vi "CTE_Analysis_Suite_UIUCv0.7.vi"() -> ()   [LabVIEW 2012]
uses:
  <vilib>/Utility/file.llb/Read From Spreadsheet File (string).vi
  <vilib>/Utility/file.llb/Write To Spreadsheet File (string).vi
panel:
  out "fpath1":string=" "
  out "deleted portion":string[][](array[string])=[["Filename", "TempC", "TempError"]]
  in  "Reset":bool
  in  "stop":bool
  in  "Tab Control":T1(tab)
  in  "iCTEAS":bool
  in  "Manual Temp Edit":bool
  in  "Remove File for Analysis":bool
  in  "Get RT Platinum Const.":bool
  out "Temperature Data from Platinum saved to:":path=path "C:/Users/jonesza/My Documents/My Dropbox/KrivenResearch/Ellipsoid/Data/testdata/CTEAS_Output/Data_Temperatures.lvm"
  in  "RT Platinum Lattice Constant":dbl=3.92296 format="%#.6g"
  in  "Load Files":bool
  in  "Input File Directory Path":path=path "C:/Users/jonesza/My Documents/My Dropbox/KrivenResearch/Ellipsoid/Data/testdata"
  out "Data Loaded":bool
  in  "Temperature Data":i32(listbox)
  in  "Input File Type":enum32{"CSV File", "JADE File"}(radio)=enum."JADE File"
  out "CTERun Path":string="C:\\Users\\jonesza\\Documents\\My Dropbox\\KrivenResearch\\Ellipsoid\\CTEAS\\data"
  in  "Crystal Symmetry":string(combo)="Monoclinic"
  in  "Phase to be Analyzed":string(combo)=" "
  in  "Polynomial Fit Order":sgl=2.0 format="%#_1g"
  out "Saved":bool
  out "File Saved to:":string="C:\\Users\\jonesza\\My Documents\\My Dropbox\\KrivenResearch\\Ellipsoid\\Data\\testdata\\CTEAS_Output\\LPTest1.csv"
  in  "Lattice Parameter Filename":string="LPTest1"
  in  "Save Lattice Parameters":bool
  in  "View Lattice Parameters":bool
  in  "gamma":bool
  in  "beta":bool
  in  "alpha":bool
  in  "c":bool
  in  "b":bool
  in  "a":bool
  out "Step 1 Data Loaded":bool
  in  "Run Analysis":bool
  in  "Symmetry\nOverride":bool
  in  "High Temperature (C)":dbl=1700.0
  in  "Temperature Step":dbl=25.0
  in  "Low Temperature (C)":dbl=25.0
  out "Results Ready":bool
  in  "HKL or UVW.":enum32{"Radio Selection 1", "Radio Selection 2"}(radio)
  in  "LW":dbl
  in  "KV":dbl=1.0
  in  "HU":dbl
  out "HU 2":string="H"
  out "KV 2":string="K"
  out "LW 2":string="L"
  in  "Make 2D Figure":bool
  in  "Make hkl (or uvw) Expansion Plot":bool
  in  "2D Figure CSV File Name":string="2Dtestfile"
  in  "Make 2D Figure CSV File":bool
  in  "Make hkl (or uvw) Expansion CSV File":bool
  in  "hkl (or uvw) Expansion CSV Filename":string="hkltestfile2"
  in  "HKL or UVW":enum32{"Radio Selection 1", "Radio Selection 2"}(radio)
  in  "hu":dbl
  out "hu":string="H"
  in  "lw":dbl=1.0
  out "lw 2":string="L"
  in  "kv":dbl
  out "kv 2":string="K"
  in  "Make CSV File":bool
  in  "CSV File Name":string="testfile"
  in  "Make Eigenvalue Plot":bool
  in  "Make 3D Figure":bool
  in  "Figure Temperature (C)":dbl=1000.0
  in  "Make Movie":bool
  in  "Movie File Name":string="testmovie"
  in  "Movie FPS":dbl=4.0
  in  "Y":dbl=768.0
  in  "X":dbl=1024.0
  out "Step 2 Analysis Run":bool
  out "BUSY":bool
  in  "Get Results":bool
  # "CTE Analysis Suite UIUC v0.61"
  # "Coefficient of Thermal Expansion Analysis Suite\nVersion: 0.6.1-Build 1\nDeveloped by: \n\n                          Zachary A. Jones\n                          Pankaj Sarin, Ph. D.\n                          Ryan P. Haggerty, Ph. D.\n\nContact Information:\n\n                          Waltraud M. Kriven, Ph. D.\n                          The University of Illinois at Urbana-Champaign\n                          Office 105 Materials Science and Engineering Building\n                          1304 W. Green St., Urbana, IL 61801\n                          Phone: (217)333-5258\n                          Fax:       (217)333-2736\n                          Email:   kriven@illinois.edu\n\n\nThis software is the intellectual property of the University of Illinois at Urbana-Champaign.  Funding for this project was provided by the Air Force Office of Scientific Research under the following grant:\n\nFA9550-06-1-0386\n\nPlease use this reference for publications including CTEAS analyses:\n\nJones, Z. 2012, \"CTEAS - A GUI based program to calculate coefficients of thermal expansion of crystalline materials from high temperature powder X-ray diffraction\", 36th International Conference & Exposition on Advanced Ceramics and Composites, Daytona Beach, FL, Hilton Daytona Beach Resort and Ocean Center, p. 41."
  # "Temperature Ranges"
  # "Lattice Parameter File Output"
  # "Lattice Parameter Selection"
  # "Select a phase first!"
  # "NOTE:\nReference angle for eigenvectors relative to hkl or uvw vector."
  # "Size of figures (in Pixels)"
  # "x"
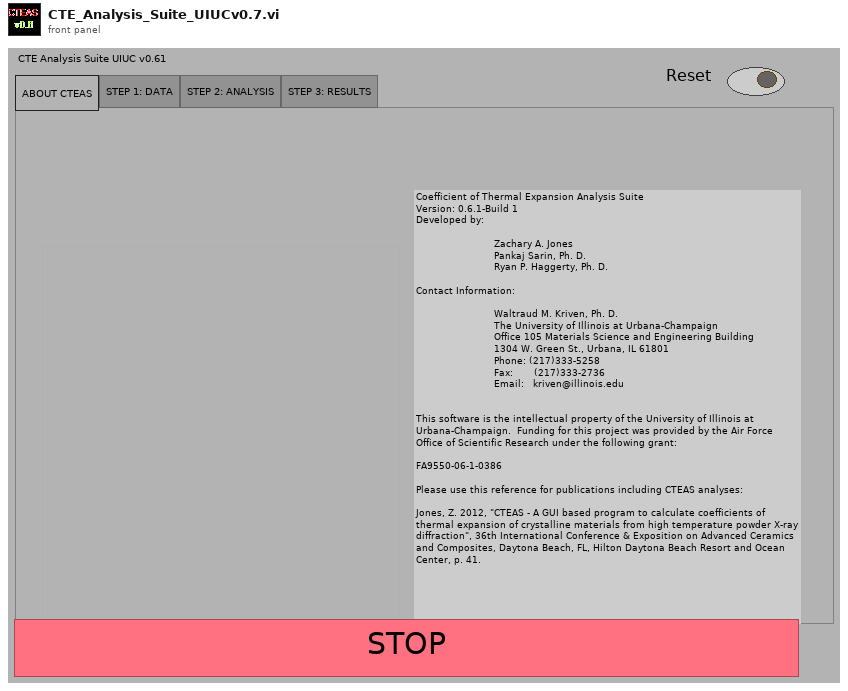
[diagram p1: front panel]
types:
  T1 = enum32{"ABOUT CTEAS", "STEP 1: DATA", "STEP 2: ANALYSIS", "STEP 3: RESULTS"}
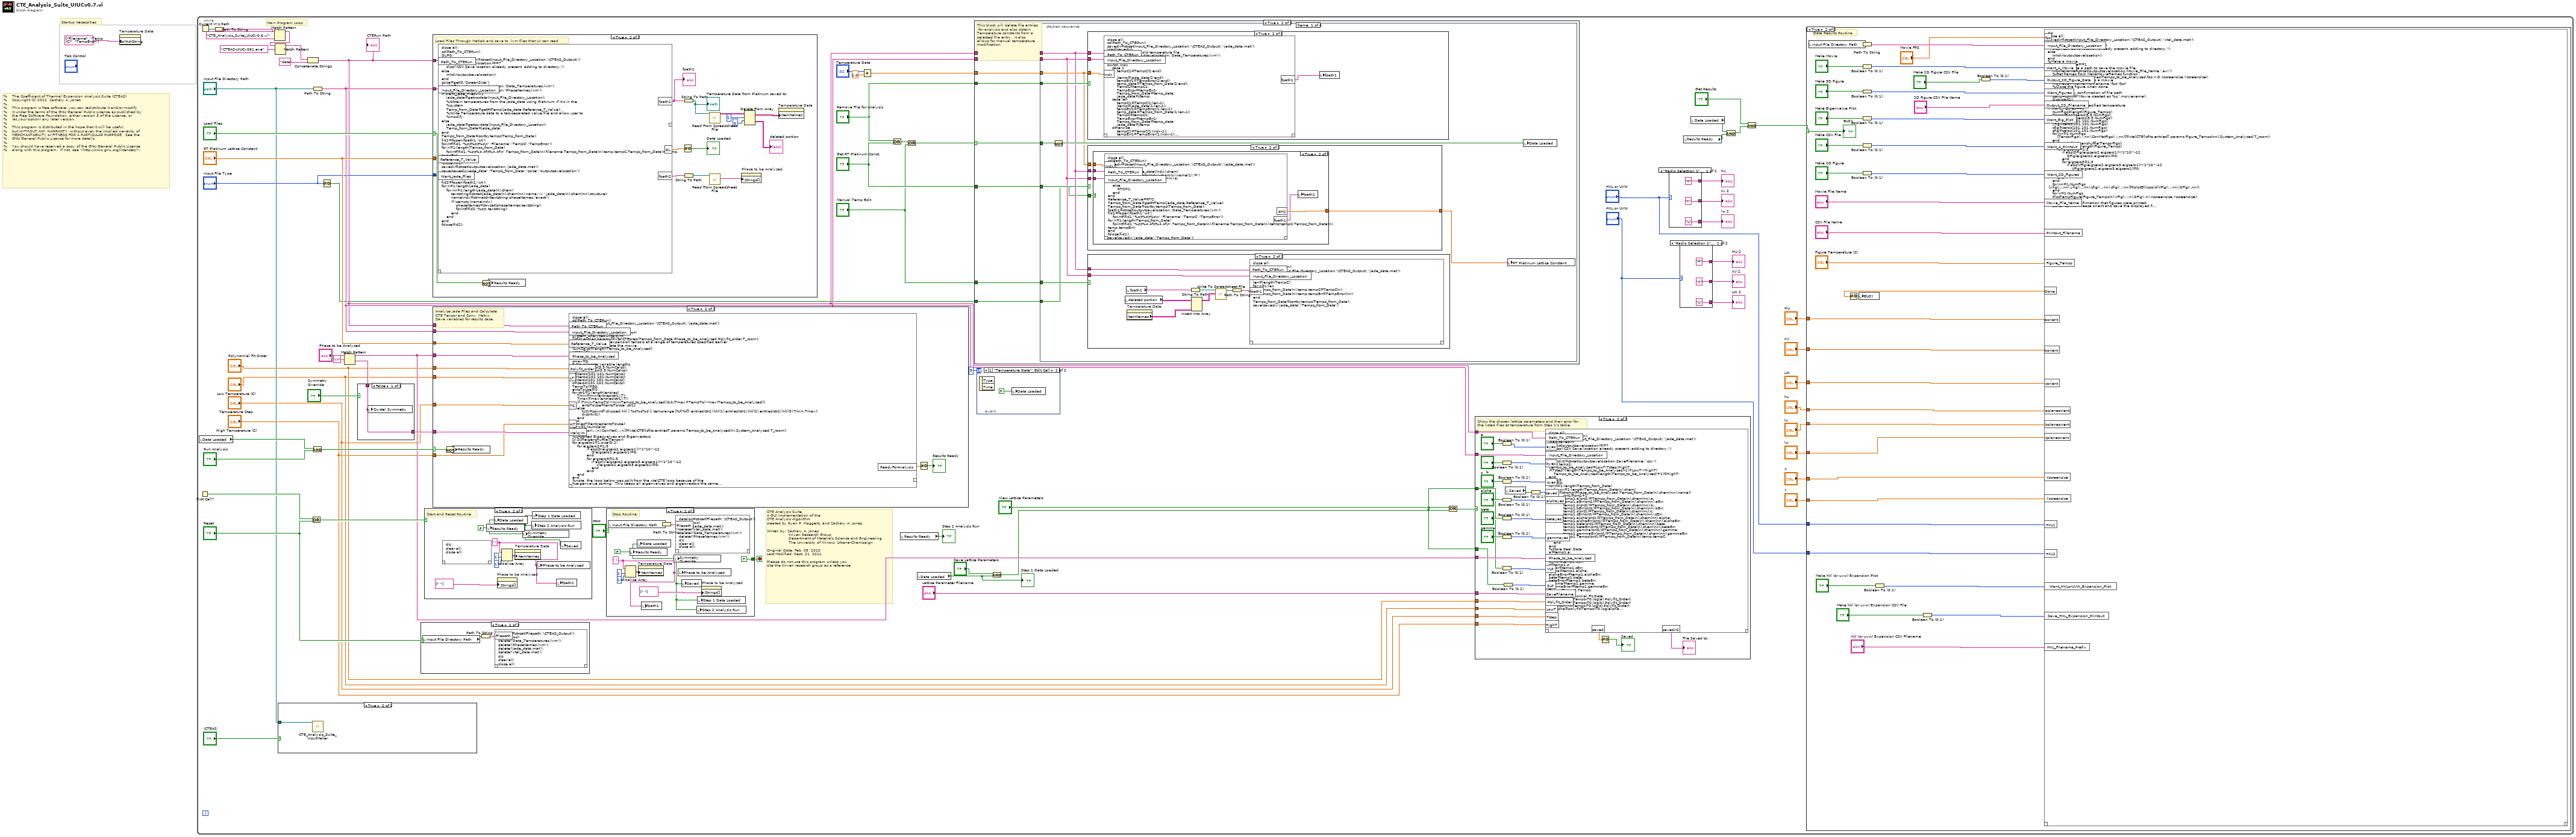
[diagram p0: block diagram]
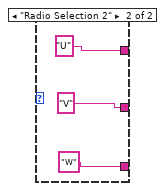
[diagram p3: hidden frame]
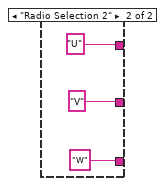
[diagram p4: hidden frame]
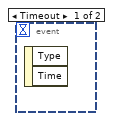
[diagram p7: hidden frame]
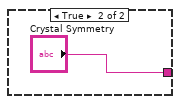
[diagram p8: hidden frame]
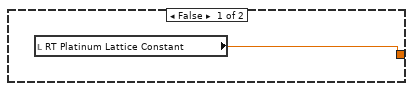
[diagram p11: hidden frame]
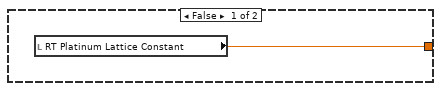
[diagram p12: hidden frame]
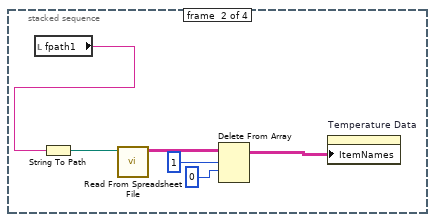
[diagram p14: hidden frame]
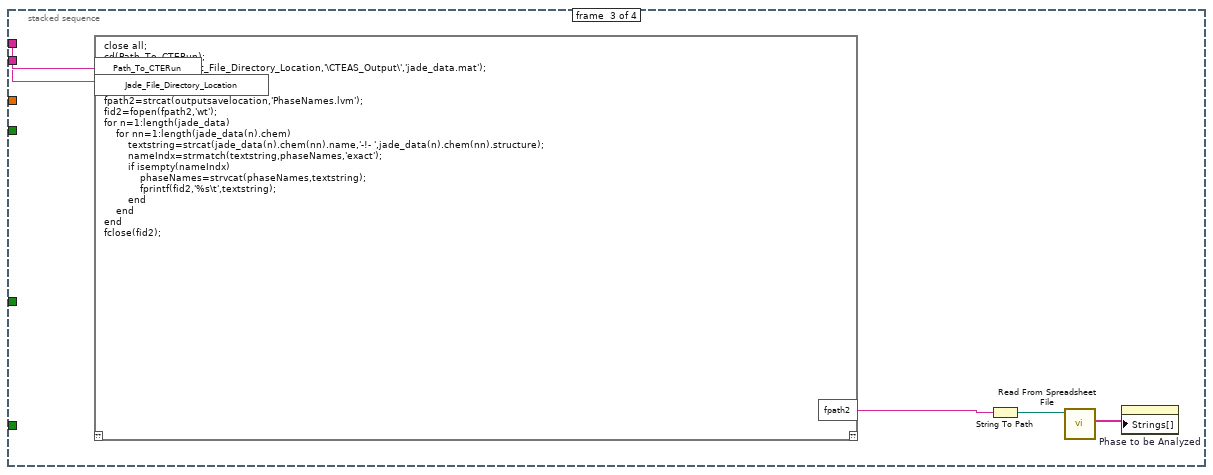
[diagram p15: hidden frame]
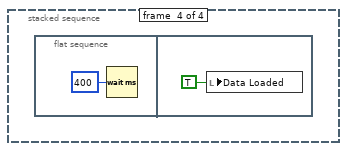
[diagram p16: hidden frame]
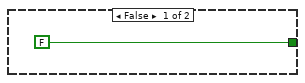
[diagram p17: hidden frame]
diagram:
  # "%    The Coefficient of Thermal Expansion Analysis Suite (CTEAS)\n%    Copyright (C) 2012  Zachary A. Jones\n%\n%    This program is free software: you can redistribute it and/or modify\n%    it under the terms of the GNU General Public License as published by\n%    the Free Software Foundation, either version 3 of the License, or\n%    (at your option) any later version.\n%\n%    This program is distributed in the hope that it will be useful,\n%    but WITHOUT ANY WARRANTY; without even the implied warranty of\n%    MERCHANTABILITY or FITNESS FOR A PARTICULAR PURPOSE.  See the\n%    GNU General Public License for more details.\n%\n%    You should have received a copy of the GNU General Public License\n%    along with this program.  If not, see <http://www.gnu.org/licenses/>."
  # "Startup Necessities"
  n1 = property on="Temperature Data" class="MCListbox (strict)"("ColHdrString"=string[] ["Filename", "Temp (C)", "TempError"]) -> ()  [unwired: 2 in, 2 out]
  n2 = while {
    stop <- w62 stop-if-true
    # "CTE Analysis Suite\nA GUI Implementation of the\nCTE Analysis Algorithm\ncreated by Ryan P. Haggerty and Zachary A. Jones.\n\nWriten by: Zachary A. Jones\n                  Kriven Research Group\n                  Department of Materials Science and Engineering\n                  The University of Illinois, Urbana-Champaign\n\nOriginal Date: Feb. 05, 2010\nLast Modified: Sept. 21, 2011\n\nPlease do not use this program unless you\ncite the Kriven research group as a reference."
    # "Main Program Loop"
    n3 = local read "Data Loaded"() -> (w69:bool)
    n4 = First Call?() -> (First Call?: T/F=w61:bool)
    n5 = Current VI's Path() -> (path=w14:path)
    n6 = Path To String(path=w14) -> (string=w11:string)
    n7 = Match Pattern(string=w11, regular expression="CTE_Analysis_Suite_UIUCv0.6.vi") -> (before substring=w8:string)  [unwired: 1 in, 3 out]
    n8 = Match Pattern(string=w8, regular expression="CTEAS-UIUCv061.exe") -> (before substring=w7:string)  [unwired: 1 in, 3 out]
    n9 = case shown="True" "iCTEAS" {
      tunnel: "Input File Directory Path" -> [_ w72]
      frame False {
      }
      frame True {
        n10 = call "CTE_Analysis_Suite_InputMaker.vi"("File Save Path"=w72) -> ()  [unwired: 11 in]
      }
    }
    n11 = Concatenate Strings(w7, "data") -> (w10:string)
    "CTERun Path" <- w10
    n12 = Or(x=w61, y="Reset") -> (x .or. y?=w60:bool)
    n13 = Path To String(path="Input File Directory Path") -> (string=w35:string)
    n14 = And(x=w69, y="Run Analysis") -> (x .and. y?=w70:bool)
    n15 = Not Equal To 0?(x="Input File Type") -> (x != 0?=w34:bool)
    n16 = Match Pattern(string="Phase to be Analyzed", regular expression="-!-") -> (before substring=w43:string, after substring=w50:string)  [unwired: 1 in, 2 out]
    n17 = case shown="False" "Symmetry\nOverride" {
      tunnel: [w117 "Crystal Symmetry"] -> w51
      tunnel: w50 -> [w117 _]
      frame False {
        n18 = local write "Crystal Symmetry"(w117) -> ()
      }
      frame True {
      }
    }
    n19 = case shown="True" "Reset" {
      frame False {
      }
      frame True {
        n20 = local read "Input File Directory Path"() -> (w85:path)
        n21 = Path To String(path=w85) -> (string=w86:string)
        n22 = script code="dataloc=strcat(Filepath,'\\CTEAS_Output');\ncd(dataloc);\ndelete('Data_Temperatures.lvm');\ndelete('PhaseNames.lvm');\ndelete('jade_data.mat');\ndelete('xtal_data.mat');\nclc;\nclear all;\nclose all;"("Filepath"=w86) -> ()  [unwired: 1 in, 1 out]
      }
    }
    n23 = case shown="True" w60 {
      frame False {
      }
      frame True {
        w222 = " "
        w223 = FALSE ("Data Loaded")
        # "Start and Reset Routine"
        n24 = script code="clc;\nclear all;\nclose all;"() -> ()  [unwired: 1 in, 1 out]
        n25 = local write "Results Ready"(w223) -> ()
        n26 = local write "Data Loaded"(w223) -> ()
        n27 = property on="Phase to be Analyzed" class="CmbBox"("Strings[]"=string[] [" "]) -> ()  [unwired: 2 in, 2 out]
        n28 = Initialize Array(w222, 1 ("dimension size"), 1 ("dimension size")) -> (w225:string[][])
        n29 = property on="Temperature Data" class="MCListbox (strict)"("ItemNames"=w225) -> ()  [unwired: 2 in, 2 out]
        n30 = local write "Symmetry\nOverride"(w223) -> ()
        n31 = local write "Step 2 Analysis Run"(w223) -> ()
        n32 = local write "Step 1 Data Loaded"(w223) -> ()
        n33 = local write "Phase to be Analyzed"(w222) -> ()
        n34 = local write "fpath1"(w222) -> ()
        n35 = local write "Saved"(w223) -> ()
      }
    }
    n36 = case shown="True" "Load Files" {
      selector: "Load Files" -> [_ w244]
      tunnel: w35 -> [_ w258]
      tunnel: w10 -> [_ w257]
      tunnel: "RT Platinum Lattice Constant" -> [_ w256]
      tunnel: "Input File Type" -> [_ w243]
      frame False {
      }
      frame True {
        # "Load Files Through Matlab and save to .lvm files that LV can read"
        n37 = script code="close all;\ncd(Path_To_CTERun);\nDL=0;\noutputsavelocation=strcat(Input_File_Directory_Location,'\\CTEAS_Output\\');\nif exist(outputsavelocation)==7\n    disp('CSV Save location already present, adding to directory.');\nelse\n    mkdir(outputsavelocation);\nend\nssize=get(0,'ScreenSize');\nfpath1=strcat(outputsavelocation,'Data_Temperatures.lvm');\nfpath2=strcat(outputsavelocation,'PhaseNames.lvm');\nif Want_Jade_Files==1\n    jade_data=getrrpdata(Input_File_Directory_Location);\n    %Obtain temperatures from the jade_data using Platinum if it's in the\n    %system\n    Temp_from_Data=getPtTemp(jade_data,Reference_T_Value);\n    %Write Temperature data to a tab-separated value file and allow user to\n    %modify.\nelse\n    jade_data=getcsvdata(Input_File_Directory_Location);\n    Temp_from_Data=jade_data;    \nend\nTemps_from_Data=sortbytemps(Temp_from_Data);\nfid1=fopen(fpath1,'wt');\nfprintf(fid1,'%s\\t%s\\t%s\\n','Filename','TempC','TempError');\nfor n=1:length(Temps_from_Data)  \n    fprintf(fid1,'%s\\t%4.4f\\t%4.4f\\n',Temps_from_Data(n).filename,Temps_from_Data(n).temp.tempC,Temps_from_Data(n).temp.tempErr);\nend\nfclose(fid1);\nsavedir=strcat(outputsavelocation,'jade_data.mat');\nsave(savedir,'jade_data','Temps_from_Data','ssize','outputsavelocation');\nDL=1;\nphaseNames={};\nfid2=fopen(fpath2,'wt');\nfor n=1:length(jade_data)\n    for nn=1:length(jade_data(n).chem)\n        textstring=strcat(jade_data(n).chem(nn).name,'-!- ',jade_data(n).chem(nn).structure);\n        nameIndx=strmatch(textstring,phaseNames,'exact');\n        if isempty(nameIndx)\n            phaseNames=strvcat(phaseNames,textstring);\n            fprintf(fid2,'%s\\t',textstring);\n        end\n    end\nend\nfclose(fid2);"("Input_File_Directory_Location"=w258, "Path_To_CTERun"=w257, "Reference_T_Value"=w256, "Want_Jade_Files"=w243) -> ("fpath1"=w241:string, "DL"=w254:dbl, "fpath2"=w242:string)  [unwired: 1 in, 1 out]
        "fpath1" <- w241
        n38 = Not(x=w244) -> (.not. x?=w245:bool)
        n39 = local write "Results Ready"(w245) -> ()
        n40 = Not Equal To 0?(x=w254) -> (x != 0?=→"Data Loaded":bool)
        n41 = String To Path(string=w241) -> (path=w255:path)
        "Temperature Data from Platinum saved to:" <- w255
        n42 = String To Path(string=w242) -> (path=w253:path)
        n43 = call-poly <vilib>:"Read From Spreadsheet File.vi"("file path (dialog if empty)"=w255) -> ("all rows"=w247:string[][])  [unwired: 6 in, 4 out]
        n44 = call-poly <vilib>:"Read From Spreadsheet File.vi"("file path (dialog if empty)"=w253) -> ("first row"=w252:string[])  [unwired: 6 in, 4 out]
        n45 = property on="Phase to be Analyzed" class="CmbBox"("Strings[]"=w252) -> ()  [unwired: 2 in, 2 out]
        n46 = Delete From Array(array=w247, length=1, index (row)=0 ("index")) -> (deleted portion=→"deleted portion":string[][], array with subset deleted=w249:string[][])  [unwired: 1 in]
        n47 = property on="Temperature Data" class="MCListbox (strict)"("ItemNames"=w249) -> ()  [unwired: 2 in, 2 out]
      }
    }
    n48 = case shown="True" w70 {
      selector: w70 -> [_ w236]
      tunnel: w10 -> [_ w240]
      tunnel: w35 -> [_ w239]
      tunnel: "RT Platinum Lattice Constant" -> [_ w238]
      tunnel: w43 -> [_ w234]
      tunnel: w51 -> [_ w233]
      tunnel: "Polynomial Fit Order" -> [_ w231]
      tunnel: "Low Temperature (C)" -> [_ w230]
      tunnel: "Temperature Step" -> [_ w229]
      tunnel: "High Temperature (C)" -> [_ w228]
      frame False {
      }
      frame True {
        # "Analyze Jade Files and Calculate\nCTE Tensor and Conv. Matrix.\nSave variables for results case."
        n49 = Not(x=w236) -> (.not. x?=w235:bool)
        n50 = local write "Results Ready"(w235) -> ()
        n51 = script code="close all;\ncd(Path_To_CTERun);\nsavedir=strcat(Input_File_Directory_Location,'\\CTEAS_Output\\','jade_data.mat');\nload(savedir);\nT_room=25;\nTemps_to_be_Analyzed=LT:TS:HT;\nSystem_Analyzed=xtalsym;\n[lsfits,entries,params]=xtalCTEprep(Temps_from_Data,Phase_to_be_Analyzed,Polyfit_order,T_room);\n%Calculate thermal expansion tensors at a range of temperatures specified earlier\n%and plot them; create the movie.\nNumCalcs=length(Temps_to_be_Analyzed);\nxmax=0;\nymax=0;\nzmax=0;\ncmax=0;\n%Pre-allocate variable lengths\nTensor=zeros(3,3,NumCalcs);\nConMat=zeros(3,3,NumCalcs);\nx=zeros(101,101,NumCalcs);\ny=zeros(101,101,NumCalcs);\nz=zeros(101,101,NumCalcs);\nc=zeros(101,101,NumCalcs);\nTempTol=50;\nentsToUse=[];\nfor ctr1=1:length(entries)\n    Tmin=min(entries(ctr1).T);\n    Tmax=max(entries(ctr1).T);\n    if (Tmin-TempTol<min(Temps_to_be_Analyzed))&&(Tmax+TempTol>max(Temps_to_be_Analyzed));\n        entsToUse=[entsToUse, ctr1];\n    else\n        txt1=sprintf('skipped hkl [ %d%d%d ], temprange [%f:%f]',entries(ctr1).hkl(1),entries(ctr1).hkl(2),entries(ctr1).hkl(3),Tmin,Tmax);\n        disp(txt1);\n    end\nend\nentriesT=entries(entsToUse);\nfor n=1:NumCalcs\n    [Tensor(:,:,n),ConMat(:,:,n)]=xtalCTE(lsfits,entriesT,params,Temps_to_be_Analyzed(n),System_Analyzed,T_room);\nend\n%Unsorted Eigenvalues and Eigenvectors\n[V,D]=eigenshuffle(Tensor);\nfor eigzero1=1:size(D,2)\n    for eigzero2=1:3\n            if abs(D(eigzero2,eigzero1))<1*10^-12\n                D(eigzero2,eigzero1)=0;\n            end\n            for eigzero3=1:3\n                if abs(V(eigzero2,eigzero3,eigzero1))<1*10^-12\n                    V(eigzero2,eigzero3,eigzero1)=0;\n                end\n            end\n    end\nend\n%note, the loop below was split from the xtalCTE loop because of the \n%eigenvalue sorting.  This keeps all eigenvalues and eigenvectors the same\n%through the calculations.\nfor n=1:NumCalcs\n    [x(:,:,n),y(:,:,n),z(:,:,n),c(:,:,n)]=plotEllipsoid(V(:,:,n),D(:,n));\nend\nsavedir=strcat(outputsavelocation,'xtal_data.mat');\nsave(savedir,'Tensor','ConMat','V','D','x','y','z','c','Temps_to_be_Analyzed','NumCalcs','System_Analyzed','lsfits','entries','entriesT','params','T_room');\nReadyForAnalysis=1;"("Path_To_CTERun"=w240, "Input_File_Directory_Location"=w239, "Reference_T_Value"=w238, "Polyfit_order"=w231, "LT"=w230, "TS"=w229, "HT"=w228, "xtalsym"=w233, "Phase_to_be_Analyzed"=w234) -> ("ReadyForAnalysis"=w237:dbl)  [unwired: 1 in, 1 out]
        n52 = Not Equal To 0?(x=w237) -> (x != 0?=→"Results Ready":bool)
      }
    }
    n53 = case shown="True" "stop" {
      tunnel: [FALSE TRUE] -> w62
      frame False {
      }
      frame True {
        w176 = " "
        w177 = FALSE
        # "Stop Routine"
        n54 = local read "Input File Directory Path"() -> (w184:path)
        n55 = Initialize Array(w176, 1 ("dimension size"), 1 ("dimension size")) -> (w180:string[][])
        n56 = local write "Results Ready"(w177) -> ()
        n57 = local write "Data Loaded"(w177) -> ()
        n58 = property on="Temperature Data" class="MCListbox (strict)"("ItemNames"=w180) -> ()  [unwired: 2 in, 2 out]
        n59 = local write "fpath1"(w176) -> ()
        n60 = Path To String(path=w184) -> (string=w183:string)
        n61 = local write "Symmetry\nOverride"(w177) -> ()
        n62 = script code="dataloc=strcat(Filepath,'\\CTEAS_Output');\ncd(dataloc);\ndelete('jade_data.mat');\ndelete('xtal_data.mat');\ndelete('Data_Temperatures.lvm');\ndelete('PhaseNames.lvm');\nclc\nclear all;\nclose all;"("Filepath"=w183) -> ()  [unwired: 1 in, 1 out]
        n63 = local write "Phase to be Analyzed"(w176) -> ()
        n64 = local write "Saved"(w177) -> ()
        n65 = local write "Step 2 Analysis Run"(w177) -> ()
        n66 = local write "Step 1 Data Loaded"(w177) -> ()
        n67 = property on="Phase to be Analyzed" class="CmbBox"("Strings[]"=string[] [" "]) -> ()  [unwired: 2 in, 2 out]
      }
    }
    n68 = Add(x="Temperature Data", y=1.0) -> (x+y=w55:dbl)
    n69 = Or(x="Remove File for Analysis", y="Get RT Platinum Const.") -> (x .or. y?=w48:bool)
    n70 = local read "Results Ready"() -> (→"Step 2 Analysis Run":bool)
    n71 = Or(x=w48, y="Manual Temp Edit") -> (x .or. y?=w47:bool)
    n72 = local read "Data Loaded"() -> (w41:bool)
    "Step 1 Data Loaded" <- w41
    n73 = case shown="True" w47 {
      selector: w47 -> [_ w123]
      tunnel: w55 -> [_ w126]
      tunnel: w10 -> [_ w122]
      tunnel: w35 -> [_ w121]
      tunnel: "Remove File for Analysis" -> [_ w125]
      tunnel: "Get RT Platinum Const." -> [_ w124]
      tunnel: "Manual Temp Edit" -> [_ w120]
      tunnel: w34 -> [_ w119]
      frame False {
      }
      frame True {
        # "This block will delete file entries\n for analysis and also obtain \nTemperature constants from a\nselected file entry.  It also\nallows for manual temperature\nmodification."
        n74 = stacked-sequence {
          tunnel: w126 -> [w133 _ _ _]
          tunnel: w125 -> [w136 _ _ _]
          tunnel: w124 -> [w129 _ _ _]
          tunnel: w123 -> [w135 _ _ _]
          tunnel: w121 -> [w130 _ w168 _]
          tunnel: w122 -> [w131 _ w169 _]
          tunnel: w120 -> [w132 _ _ _]
          tunnel: w119 -> [w128 _ _ _]
          frame #0 {
            n75 = Not(x=w135) -> (.not. x?=w134:bool)
            n76 = case shown="True" w136 {
              tunnel: w133 -> [_ w161]
              tunnel: w131 -> [_ w160]
              tunnel: w130 -> [_ w159]
              frame False {
              }
              frame True {
                n77 = script code="close all;\ncd(Path_To_CTERun);\nsavedir=strcat(Input_File_Directory_Location,'\\CTEAS_Output\\','jade_data.mat');\nload(savedir);\n%Get Temps from old temperature file\nfpath1=strcat(outputsavelocation,'Data_Temperatures.lvm');\ntdfread(fpath1,'\\t');\nlen=length(TempC);\nswitch Indx\n    case 1\n        tempC1=TempC(2:end);\n\n        jtemp=jade_data(2:end);\n        tempErr1=TempError(2:end);\n        temp_data=Temps_from_Data(2:end);\n        TempC=tempC1;\n        TempError=tempErr1;\n        Temps_from_Data=temp_data;\n        jade_data=jtemp;\n    case len\n        tempC1=TempC(1:len-1);\n        jtemp=jade_data(1:len-1);\n        tempErr1=TempError(1:len-1);\n        temp_data=Temps_from_Data(1:len-1);\n        TempC=tempC1;\n        TempError=tempErr1;\n        Temps_from_Data=temp_data;\n        jade_data=jtemp;\n    otherwise\n        tempC1=TempC(1:Indx-1);\n        tempErr1=TempError(1:Indx-1);\n        temp_data=Temps_from_Data(1:Indx-1);\n        tempC2=TempC(Indx+1:end);\n        tempErr2=TempError(Indx+1:end);\n        jtemp1=jade_data(1:Indx-1);\n        jtemp2=jade_data(Indx+1:end);\n        temp_data2=Temps_from_Data(Indx+1:end);\n        clear TempC;\n        clear TempError;\n        clear Temps_from_Data;\n        clear jade_data;\n        for nn=1:length(tempC1)\n            TempC(nn)=tempC1(nn);\n            TempError(nn)=tempErr1(nn);\n            Temps_from_Data(nn)=temp_data(nn);\n            jade_data(nn)=jtemp1(nn);\n        end\n        ctr=1;\n        for nnn=nn+1:length(tempC2)+nn\n            TempC(nnn)=tempC2(ctr);\n            TempError(nnn)=tempErr2(ctr);\n            Temps_from_Data(nnn)=temp_data2(ctr);\n            jade_data(nnn)=jtemp2(ctr);\n            ctr=ctr+1;\n        end\nend\nfor nn=1:length(Temps_from_Data)\n    Temps_from_Data(nn).temp.tempC=TempC(nn);\n    Temps_from_Data(nn).temp.tempErr=TempError(nn);\nend\n\nTemps_from_Data=sortbytemps(Temps_from_Data);\ndelete(fpath1);\nfid1=fopen(fpath1,'wt');\n    fprintf(fid1,'%s\\t%s\\t%s\\n','Filename','TempC','TempError');\nfor n=1:length(Temps_from_Data)  \n    fprintf(fid1,'%s\\t%4.4f\\t%4.4f\\n',Temps_from_Data(n).filename,Temps_from_Data(n).temp.tempC,Temps_from_Data(n).temp.tempErr);\nend\nfclose(fid1);\nsave(savedir,'jade_data','Temps_from_Data');"("Indx"=w161, "Path_To_CTERun"=w160, "Input_File_Directory_Location"=w159) -> ("fpath1"=w158:string)  [unwired: 1 in, 1 out]
                n78 = local write "fpath1"(w158) -> ()
              }
            }
            n79 = case shown="True" w128 {
              tunnel: [w146 w151] -> w127
              tunnel: w131 -> [_ w150]
              tunnel: w130 -> [_ w149]
              tunnel: w133 -> [_ w148]
              tunnel: w129 -> [_ w147]
              frame False {
                n80 = local read "RT Platinum Lattice Constant"() -> (w146:dbl)
              }
              frame True {
                n81 = case shown="True" w147 {
                  tunnel: [w152 w157] -> w151
                  tunnel: w150 -> [_ w156]
                  tunnel: w149 -> [_ w155]
                  tunnel: w148 -> [_ w154]
                  frame False {
                    n82 = local read "RT Platinum Lattice Constant"() -> (w152:dbl)
                  }
                  frame True {
                    n83 = script code="close all;\ncd(Path_To_CTERun);\nsavedir=strcat(Input_File_Directory_Location,'\\CTEAS_Output\\','jade_data.mat');\nload(savedir);\nfor n=1:length(jade_data(Indx).chem)\n    if strcmp(jade_data(Indx).chem(n).name(1),'P')\n        RTC=jade_data(Indx).chem(n).a;\n        break;\n    else\n        RTC=1;\n    end\nend\nReference_T_Value=RTC;\nTemps_from_Data=getPtTemp(jade_data,Reference_T_Value);\nTemps_from_Data=sortbytemps(Temps_from_Data);\nfpath1=strcat(outputsavelocation,'Data_Temperatures.lvm');\nfid1=fopen(fpath1,'wt');\n    fprintf(fid1,'%s\\t%s\\t%s\\n','Filename','TempC','TempError');\nfor n=1:length(Temps_from_Data)  \n    fprintf(fid1,'%s\\t%4.4f\\t%4.4f\\n',Temps_from_Data(n).filename,Temps_from_Data(n).temp.tempC,Temps_from_Data(n).temp.tempErr);\nend\nfclose(fid1);\nsave(savedir,'jade_data','Temps_from_Data');"("Indx"=w154, "Path_To_CTERun"=w156, "Input_File_Directory_Location"=w155) -> ("RTC"=w157:dbl, "fpath1"=w153:string)  [unwired: 1 in, 1 out]
                    n84 = local write "fpath1"(w153) -> ()
                  }
                }
              }
            }
            n85 = case shown="True" w132 {
              tunnel: w130 -> [_ w137]
              tunnel: w131 -> [_ w138]
              frame False {
              }
              frame True {
                n86 = local read "deleted portion"() -> (w143:string[][])
                n87 = local read "fpath1"() -> (w145:string)
                n88 = property on="Temperature Data" class="MCListbox (strict)"() -> ("ItemNames"=w142:string[][])  [unwired: 2 in, 2 out]
                n89 = String To Path(string=w145) -> (path=w144:path)
                n90 = Insert Into Array(array=w143, new element=w142) -> (w141:string[][])  [unwired: 2 in]
                n91 = call-poly <vilib>:"Write To Spreadsheet File.vi"("2D data"=w141, "file path (dialog if empty)"=w144) -> ("new file path (Not A Path if cancelled)"=w140:path)  [unwired: 6 in]
                n92 = Path To String(path=w140) -> (string=w139:string)
                n93 = script code="close all;\ncd(Path_To_CTERun);\nsavedir=strcat(Input_File_Directory_Location,'\\CTEAS_Output\\','jade_data.mat');\nload(savedir);\ntdfread(fpath1,'\\t');\nlen=length(TempC);\nfor n=1:len\n    Temps_from_Data(n).temp.tempC=TempC(n);\n    Temps_from_Data(n).temp.tempErr=TempError(nn);\nend\nTemps_from_Data=sortbytemps(Temps_from_Data);\nsave(savedir,'jade_data','Temps_from_Data');"("fpath1"=w139, "Path_To_CTERun"=w138, "Input_File_Directory_Location"=w137) -> ()  [unwired: 1 in, 1 out]
              }
            }
            n94 = local write "RT Platinum Lattice Constant"(w127) -> ()
            n95 = local write "Data Loaded"(w134) -> ()
          }
          frame #1 {
            n96 = local read "fpath1"() -> (w162:string)
            n97 = String To Path(string=w162) -> (path=w166:path)
            n98 = call-poly <vilib>:"Read From Spreadsheet File.vi"("file path (dialog if empty)"=w166) -> ("all rows"=w167:string[][])  [unwired: 6 in, 4 out]
            n99 = Delete From Array(array=w167, length=1, index (row)=0 ("index")) -> (array with subset deleted=w163:string[][])  [unwired: 1 in, 1 out]
            n100 = property on="Temperature Data" class="MCListbox (strict)"("ItemNames"=w163) -> ()  [unwired: 2 in, 2 out]
          }
          frame #2 {
            n101 = script code="close all;\ncd(Path_To_CTERun);\nsavedir=strcat(Input_File_Directory_Location,'\\CTEAS_Output\\','jade_data.mat');\nload(savedir);\nphaseNames={};\nfpath2=strcat(outputsavelocation,'PhaseNames.lvm');\nfid2=fopen(fpath2,'wt');\nfor n=1:length(jade_data)\n    for nn=1:length(jade_data(n).chem)\n        textstring=strcat(jade_data(n).chem(nn).name,'-!- ',jade_data(n).chem(nn).structure);\n        nameIndx=strmatch(textstring,phaseNames,'exact');\n        if isempty(nameIndx)\n            phaseNames=strvcat(phaseNames,textstring);\n            fprintf(fid2,'%s\\t',textstring);\n        end\n    end\nend\nfclose(fid2);"("Path_To_CTERun"=w169, "Jade_File_Directory_Location"=w168) -> ("fpath2"=w170:string)  [unwired: 1 in, 1 out]
            n102 = String To Path(string=w170) -> (path=w172:path)
            n103 = call-poly <vilib>:"Read From Spreadsheet File.vi"("file path (dialog if empty)"=w172) -> ("first row"=w171:string[])  [unwired: 6 in, 4 out]
            n104 = property on="Phase to be Analyzed" class="CmbBox"("Strings[]"=w171) -> ()  [unwired: 2 in, 2 out]
          }
          frame #3 {
            n105 = flat-sequence {
              frame #0 {
                n106 = Wait (ms)(milliseconds to wait=u32 400) -> ()  [unwired: 1 out]
              }
              frame #1 {
                n107 = local write "Data Loaded"(TRUE) -> ()
              }
            }
          }
        }
      }
    }
    n108 = event shown="[1] \"Temperature Data\": Edit Cell" {
      selector: _ -> [_ _]
      dyn-events: _ -> [_ _]
      timeout: 3 -> [_ _]
      event Timeout {
        n109 = event-data() -> ()  [unwired: 1 in, 2 out]
      }
      event "Temperature Data": Edit Cell {
        n110 = event-data() -> ()  [unwired: 1 in, 2 out]
        n111 = local write "Data Loaded"(FALSE) -> ()
      }
    }
    n112 = And(x="Save Lattice Parameters", y=w41) -> (x .and. y?=w36:bool)
    n113 = Or(x="View Lattice Parameters", y=w36) -> (x .or. y?=w39:bool)
    n114 = case shown="True" w39 {
      tunnel: w35 -> [_ w114]
      tunnel: w10 -> [_ w115]
      tunnel: w43 -> [_ w101]
      tunnel: "View Lattice Parameters" -> [_ w99]
      tunnel: "Lattice Parameter Filename" -> [_ w97]
      tunnel: w36 -> [_ w93]
      tunnel: "Polynomial Fit Order" -> [_ w90]
      tunnel: "Low Temperature (C)" -> [_ w89]
      tunnel: "Temperature Step" -> [_ w88]
      tunnel: "High Temperature (C)" -> [_ w87]
      frame False {
      }
      frame True {
        # "Show the chosen lattice parameters and their error for\nthe listed files at temperature from Step 1's table."
        n115 = Boolean To (0,1)(Boolean="a") -> (0, 1=w112:i16)
        n116 = Boolean To (0,1)(Boolean="b") -> (0, 1=w110:i16)
        n117 = Boolean To (0,1)(Boolean="c") -> (0, 1=w108:i16)
        n118 = Boolean To (0,1)(Boolean="alpha") -> (0, 1=w106:i16)
        n119 = Boolean To (0,1)(Boolean="beta") -> (0, 1=w104:i16)
        n120 = Boolean To (0,1)(Boolean="gamma") -> (0, 1=w102:i16)
        n121 = Boolean To (0,1)(Boolean=w99) -> (0, 1=w100:i16)
        n122 = Boolean To (0,1)(Boolean=w93) -> (0, 1=w98:i16)
        n123 = local read "Saved"() -> (w91:bool)
        n124 = Boolean To (0,1)(Boolean=w91) -> (0, 1=w92:i16)
        n125 = script code="close all;\ncd(Path_To_CTERun);\nsavedir=strcat(Input_File_Directory_Location,'\\CTEAS_Output\\','jade_data.mat');\nload(savedir);\nif exist(outputsavelocation)==7\n    disp('CSV Save location already present, adding to directory.');\nelse\n    mkdir(outputsavelocation);\nend\nsavedir2=strcat(outputsavelocation,SaveFilename,'.csv');\nclear temp1;\nTemps_to_be_Analyzed=LowT:Tstep:HighT;\nif(Tstep*(length(Temps_to_be_Analyzed)-1)+LowT<HighT)\n    Temps_to_be_Analyzed(length(Temps_to_be_Analyzed)+1)=HighT;\nend\nT0=25;\ncnt1=0;\nfor n=1:length(Temps_from_Data)\n    for nn=1:length(Temps_from_Data(n).chem)\n        if(strcmp(Phase_to_be_Analyzed,Temps_from_Data(n).chem(nn).name))\n            cnt1=cnt1+1\n            temp1.a(cnt1)=Temps_from_Data(n).chem(nn).a;\n            temp1.aErr(cnt1)=Temps_from_Data(n).chem(nn).aErr;\n            temp1.b(cnt1)=Temps_from_Data(n).chem(nn).b;\n            temp1.bErr(cnt1)=Temps_from_Data(n).chem(nn).bErr;\n            temp1.c(cnt1)=Temps_from_Data(n).chem(nn).c;\n            temp1.cErr(cnt1)=Temps_from_Data(n).chem(nn).cErr;\n            temp1.alpha(cnt1)=Temps_from_Data(n).chem(nn).alpha;\n            temp1.alphaErr(cnt1)=Temps_from_Data(n).chem(nn).alphaErr;\n            temp1.beta(cnt1)=Temps_from_Data(n).chem(nn).beta;\n            temp1.betaErr(cnt1)=Temps_from_Data(n).chem(nn).betaErr;\n            temp1.gamma(cnt1)=Temps_from_Data(n).chem(nn).gamma;\n            temp1.gammaErr(cnt1)=Temps_from_Data(n).chem(nn).gammaErr;\n            temp1.Temps(cnt1)=Temps_from_Data(n).temp.tempC;\n        end\n    end\nend\n%Store Real Data\na=temp1.a;\naError=temp1.aErr;\nb=temp1.b;\nbError=temp1.bErr;\nc=temp1.c;\ncError=temp1.cErr;\nalpha=temp1.alpha;\nalphaError=temp1.alphaErr;\nbeta=temp1.beta;\nbetaError=temp1.betaErr;\ngamma=temp1.gamma;\ngammaError=temp1.gammaErr;\nTemps=temp1.Temps;\n\n%Create Polynomial Fit Data\nfitsa=polyfit(Temps-T0,log(a),Polyfit_Order);\nfitsb=polyfit(Temps-T0,log(b),Polyfit_Order);\nfitsc=polyfit(Temps-T0,log(c),Polyfit_Order);\nfitsalpha=polyfit(Temps-T0,log(alpha),Polyfit_Order);\nfitsbeta=polyfit(Temps-T0,log(beta),Polyfit_Order);\nfitsgamma=polyfit(Temps-T0,log(gamma),Polyfit_Order);\n%Zero out some arrays:\nfitlinesa=zeros(length(Temps_to_be_Analyzed),1);\nfitlinesb=zeros(length(Temps_to_be_Analyzed),1);\nfitlinesc=zeros(length(Temps_to_be_Analyzed),1);\nfitlinesalpha=zeros(length(Temps_to_be_Analyzed),1);\nfitlinesbeta=zeros(length(Temps_to_be_Analyzed),1);\nfitlinesgamma=zeros(length(Temps_to_be_Analyzed),1);\nfitlinesad=zeros(length(Temps),1);\nfitlinesbd=zeros(length(Temps),1);\nfitlinescd=zeros(length(Temps),1);\nfitlinesalphad=zeros(length(Temps),1);\nfitlinesbetad=zeros(length(Temps),1);\nfitlinesgammad=zeros(length(Temps),1);\n\n%Create Fitted Lattice Parameter Values\nfor n=1:length(Temps_to_be_Analyzed)\n    T1=Temps_to_be_Analyzed(n);\n    %Obtain a fitted lattice parameter at a given temperature\n    fitlinesa(n)=fitlinesa(n)+polyval(fitsa,T1-T0);\n    fitlinesb(n)=fitlinesb(n)+polyval(fitsb,T1-T0);\n    fitlinesc(n)=fitlinesc(n)+polyval(fitsc,T1-T0);\n    fitlinesalpha(n)=fitlinesalpha(n)+polyval(fitsalpha,T1-T0);\n    fitlinesbeta(n)=fitlinesbeta(n)+polyval(fitsbeta,T1-T0);\n    fitlinesgamma(n)=fitlinesgamma(n)+polyval(fitsgamma,T1-T0);\nend\n\n%Clean up by making sure we have exp(fit) instead of an ln fit.\nfitlines.a=exp(fitlinesa);\nfitlines.b=exp(fitlinesb);\nfitlines.c=exp(fitlinesc);\nfitlines.alpha=exp(fitlinesalpha);\nfitlines.beta=exp(fitlinesbeta);\nfitlines.gamma=exp(fitlinesgamma);\n\n%Calculate Coefficient of Determination:\n%Now calculate coefficient of determination:\nfor n=1:length(Temps)\n    T1=Temps(n);\n    fitlinesad(n)=exp(polyval(fitsa,T1-T0));\n    aresid(n)=a(n)-fitlinesad(n);\n    fitlinesbd(n)=exp(polyval(fitsb,T1-T0));\n    bresid(n)=b(n)-fitlinesbd(n);\n    fitlinescd(n)=exp(polyval(fitsc,T1-T0));\n    cresid(n)=c(n)-fitlinescd(n);\n    fitlinesalphad(n)=exp(polyval(fitsalpha,T1-T0));\n    alpharesid(n)=alpha(n)-fitlinesalphad(n);\n    fitlinesbetad(n)=exp(polyval(fitsbeta,T1-T0));\n    betaresid(n)=beta(n)-fitlinesbetad(n);\n    fitlinesgammad(n)=exp(polyval(fitsgamma,T1-T0));\n    gammaresid(n)=gamma(n)-fitlinesgammad(n);\nend\nSSaresid=sum(aresid.^2);\nSSbresid=sum(bresid.^2);\nSScresid=sum(cresid.^2);\nSSalpharesid=sum(alpharesid.^2);\nSSbetaresid=sum(betaresid.^2);\nSSgammaresid=sum(gammaresid.^2);    \nSSatotal=(length(a)-1)*var(a);\nSSbtotal=(length(b)-1)*var(b);\nSSctotal=(length(c)-1)*var(c);\nSSalphatotal=(length(alpha)-1)*var(alpha);\nSSbetatotal=(length(beta)-1)*var(beta);\nSSgammatotal=(length(gamma)-1)*var(gamma);\nrsqa=1-(SSaresid/SSatotal);\nrsqb=1-(SSbresid/SSbtotal);\nrsqc=1-(SScresid/SSctotal);\nrsqalpha=1-(SSalpharesid/SSalphatotal);\nrsqbeta=1-(SSbetaresid/SSbetatotal);\nrsqgamma=1-(SSgammaresid/SSgammatotal);\nresiduals.Ra=rsqa;\nresiduals.Rb=rsqb;\nresiduals.Rc=rsqc;\nresiduals.Ralpha=rsqalpha;\nresiduals.Rbeta=rsqbeta;\nresiduals.Rgamma=rsqgamma;\n    \nif VLP==1\n    ssize=get(0,'ScreenSize');\n    latlegend={};\n    ctr1=1;\n    ctr2=1;\n    anglegend={};\n    if ayes==1 || byes==1 || cyes==1\n        k=figure('Position',[((ssize(3)/2)-(ssize(3)*3/8)) ((ssize(4)/2)-(ssize(4)*3/8)) ssize(3)*.75 ssize(4)*.75]);\n        if ayes==1\n            errorbar(Temps,a,aError,'bo');\n            latlegend(ctr1)={'a'};\n            ctr1=ctr1+1;\n\t\t\thold on;\n\t\t\tplot(Temps_to_be_Analyzed,fitlines.a,'b:');\n\t\t\tlegnamea=strcat('Fit a, R^2=',num2str(residuals.Ra));\n\t\t\tlatlegend(ctr1)={legnamea};\n\t\t\tctr1=ctr1+1;\n            hold on;\n        end\n        if byes==1\n            errorbar(Temps,b,bError,'ro');\n            latlegend(ctr1)={'b'};\n            ctr1=ctr1+1;\n\t\t\thold on;\n\t\t\tplot(Temps_to_be_Analyzed,fitlines.b,'r:');\n\t\t\tlegnameb=strcat('Fit b, R^2=',num2str(residuals.Rb));\n\t\t\tlatlegend(ctr1)={legnameb};\n\t\t\tctr1=ctr1+1;\n            hold on;\n        end\n        if cyes==1\n            errorbar(Temps,c,cError,'ko');\n            latlegend(ctr1)={'c'};\n\t\t\tctr1=ctr1+1;\n\t\t\thold on;\n\t\t\tplot(Temps_to_be_Analyzed,fitlines.c,'k:');\n\t\t\tlegnamec=strcat('Fit c, R^2=',num2str(residuals.Rc));\n\t\t\tlatlegend(ctr1)={legnamec};\n            hold on;\n        end\n        xscreen=ssize(3)*0.75;\n        yscreen=ssize(4)*0.75;\n        fontsize=round(xscreen/85);\n        if(fontsize<12)\n            fontsize=12;\n        end\n        titlesize=round(xscreen/50);\n        if(titlesize<20)\n            titlesize=20;\n        end\n        title('Lattice Parameters vs. Temperature','FontSize',titlesize,'FontWeight','bold');\n        xlabel(strcat('Temperature (',char(176),'C)'),'FontSize',fontsize);\n        ylabel(strcat('Lattice Parameters (',char(197),')'),'Fontsize',fontsize);\n        legend(latlegend);\n        set(gca,'FontSize',fontsize);\n        hold off;\n    end\n    if alphayes==1 || betayes==1 || gammayes==1\n        l=figure('Position',[((ssize(3)/2)-(ssize(3)*3/8)) ((ssize(4)/2)-(ssize(4)*3/8)) ssize(3)*.75 ssize(4)*.75]);\n        if alphayes==1\n            errorbar(Temps,alpha,alphaError,'bo');\n            anglegend(ctr2)={'alpha'};\n            ctr2=ctr2+1;\n            hold on;\n\t\t\tplot(Temps_to_be_Analyzed,fitlines.alpha,'b:');\n\t\t\tlegnamealpha=strcat('Fit alpha, R^2=',num2str(residuals.Ralpha));\n\t\t\tanglegend(ctr2)={legnamealpha};\n\t\t\tctr2=ctr2+1;\n            hold on;\n        end\n        if betayes==1\n            errorbar(Temps,beta,betaError,'ro');\n            anglegend(ctr2)={'beta'};\n            ctr2=ctr2+1;\n            hold on;\n\t\t\tplot(Temps_to_be_Analyzed,fitlines.beta,'r:');\n\t\t\tlegnamebeta=strcat('Fit beta, R^2=',num2str(residuals.Rbeta));\n\t\t\tanglegend(ctr2)={legnamebeta};\n\t\t\tctr2=ctr2+1;\n            hold on;\n        end\n        if gammayes==1\n            errorbar(Temps,gamma,gammaError,'ko');\n            anglegend(ctr2)={'gamma'};\n            hold on;\n\t\t\tctr2=ctr2+1;\n\t\t\tplot(Temps_to_be_Analyzed,fitlines.gamma,'k:');\n\t\t\tlegnamegamma=strcat('Fit gamma, R^2=',num2str(residuals.Rgamma));\n\t\t\tanglegend(ctr2)={legnamegamma};\n            hold on;\n        end\n        title('Lattice Parameter Angles vs. Temperature','FontSize',titlesize,'FontWeight','bold')\n        xlabel(strcat('Temperature (',char(176),'C)'),'FontSize',fontsize);\n        ylabel('Lattice Parameter Angles (deg.)','FontSize',fontsize);\n        legend(anglegend);\n        set(gca,'FontSize',fontsize);\n        hold off;\n    end\nend\nif SLP==1\n    fid1=fopen(savedir2,'wt');\n    fprintf(fid1,'Temp (C),a,aError,b,bError,c,cError,alpha,alphaError,beta,betaError,gamma,gammaError\\n');\n    for n=1:length(Temps)\n        fprintf(fid1,'%4.4f,%4.4f,%4.4f,%4.4f,%4.4f,%4.4f,%4.4f,%4.4f,%4.4f,%4.4f,%4.4f,%4.4f,%4.4f\\n',Temps(n),a(n),aError(n),b(n),bError(n),c(n),cError(n),alpha(n),alphaError(n),beta(n),betaError(n),gamma(n),gammaError(n));\n    end\n    fclose(fid1);\n    saved=1;\nend"("Path_To_CTERun"=w115, "Input_File_Directory_Location"=w114, "ayes"=w112, "byes"=w110, "cyes"=w108, "alphayes"=w106, "betayes"=w104, "gammayes"=w102, "Phase_to_be_Analyzed"=w101, "VLP"=w100, "SLP"=w98, "SaveFilename"=w97, "saved"=w92, "Polyfit_Order"=w90, "LowT"=w89, "Tstep"=w88, "HighT"=w87) -> ("savedir2"=→"File Saved to:":string, "saved"=w95:dbl)  [unwired: 1 in, 1 out]
        n126 = Not Equal To 0?(x=w95) -> (x != 0?=→"Saved":bool)
      }
    }
    n127 = case shown="\"Radio Selection 1\", Default" "HKL or UVW" {
      tunnel: ["H" "U"] -> w26
      tunnel: ["K" "V"] -> w31
      tunnel: ["L" "W"] -> w30
      frame "Radio Selection 1", Default {
      }
      frame "Radio Selection 2" {
      }
    }
    "hu" <- w26
    "kv 2" <- w31
    "lw 2" <- w30
    n128 = case shown="\"Radio Selection 1\", Default" "HKL or UVW." {
      tunnel: ["H" "U"] -> w29
      tunnel: ["K" "V"] -> w28
      tunnel: ["L" "W"] -> w27
      frame "Radio Selection 1", Default {
      }
      frame "Radio Selection 2" {
      }
    }
    "HU 2" <- w29
    "KV 2" <- w28
    "LW 2" <- w27
    n129 = local read "Results Ready"() -> (w64:bool)
    n130 = local read "Data Loaded"() -> (w65:bool)
    n131 = And(x=w65, y=w64) -> (x .and. y?=w67:bool)
    n132 = And(x="Get Results", y=w67) -> (x .and. y?=w63:bool)
    n133 = case shown="True" w63 {
      selector: w63 -> [_ w206]
      tunnel: "HKL or UVW" -> [_ w203]
      tunnel: "HKL or UVW." -> [_ w202]
      tunnel: "HU" -> [_ w199]
      tunnel: "KV" -> [_ w198]
      tunnel: "LW" -> [_ w197]
      tunnel: "hu" -> [_ w196]
      tunnel: "kv" -> [_ w195]
      tunnel: "lw" -> [_ w194]
      tunnel: "X" -> [_ w193]
      tunnel: "Y" -> [_ w192]
      frame False {
      }
      frame True {
        # "Data Results Routine"
        n134 = local read "Input File Directory Path"() -> (w217:path)
        n135 = Path To String(path=w217) -> (string=w216:string)
        n136 = Boolean To (0,1)(Boolean="Make Movie") -> (0, 1=w215:i16)
        n137 = Boolean To (0,1)(Boolean="Make 3D Figure") -> (0, 1=w214:i16)
        n138 = Boolean To (0,1)(Boolean="Make Eigenvalue Plot") -> (0, 1=w213:i16)
        n139 = Boolean To (0,1)(Boolean="Make CSV File") -> (0, 1=w211:i16)
        n140 = Boolean To (0,1)(Boolean="Make 2D Figure") -> (0, 1=w212:i16)
        n141 = Boolean To (0,1)(Boolean="Make hkl (or uvw) Expansion Plot") -> (0, 1=w200:i16)
        n142 = Boolean To (0,1)(Boolean="Make hkl (or uvw) Expansion CSV File") -> (0, 1=w187:i16)
        n143 = Boolean To (0,1)(Boolean="Make 2D Figure CSV File") -> (0, 1=w190:i16)
        n144 = script code="clc;\nclose all;\nsavedir=strcat(Input_File_Directory_Location,'\\CTEAS_Output\\','xtal_data.mat');\nload(savedir);\nif exist(outputsavelocation)==7\n    disp('CSV Save location already present, adding to directory.');\nelse\n    mkdir(outputsavelocation);\nend\n%Make a movie\nif Want_A_Movie==1\n    %Concatenate a path to save the movie file.\n    moviename=strcat(outputsavelocation,Movie_File_Name,'.avi');\n    %Get frames from MakeMovieFrames function\n    frame=MakeMovieFrames(Temps_to_be_Analyzed,fps,V,D,Xscreensize,Yscreensize);\n    %Convert the frames to a movie\n    movie2avi(frame,moviename,'fps',fps)\n    %Close the figure when done.\n    close all;\n    %Obligatory confirmation of file path\n    part1=sprintf('Movie created as %s.',moviename);\n    disp(part1);\nend\n%Plot figure(s) at a specified temperature\nif Want_Figures==1\n    NumFigs=length(Figure_Temps);\n    TensorFigs=zeros(3,3,NumFigs);\n    ConMatFigs=zeros(3,3,NumFigs);\n    xfig=zeros(101,101,NumFigs);\n    yfig=zeros(101,101,NumFigs);\n    zfig=zeros(101,101,NumFigs);\n    cfig=zeros(101,101,NumFigs);\n    for nn=1:NumFigs\n        [TensorFigs(:,:,nn),ConMatFigs(:,:,nn)]=xtalCTE(lsfits,entriesT,params,Figure_Temps(nn),System_Analyzed,T_room);\n    end\n    [VFig,DFig]=eigenshuffle(TensorFigs);\n    for eigzero1=1:length(Figure_Temps)\n        for eigzero2=1:3\n            if abs(DFig(eigzero2,eigzero1))<1*10^-12\n                DFig(eigzero2,eigzero1)=0;\n            end\n            for eigzero3=1:3\n                if abs(VFig(eigzero2,eigzero3,eigzero1))<1*10^-12\n                    VFig(eigzero2,eigzero3,eigzero1)=0;\n                end\n            end            \n        end\n    end\n    for nn=1:NumFigs\n\t[xfig(:,:,nn),yfig(:,:,nn),zfig(:,:,nn),cfig(:,:,nn)]=plotEllipsoid(VFig(:,:,nn),DFig(:,nn));\n    end\n    for n=1:NumFigs\n    PlotTempFigure(Figure_Temps(n),VFig(:,:,n),DFig(:,n),Xscreensize,Yscreensize);\n    end\n    %Obligitory confirmation that figures were printed.\n    part2=sprintf('Please orient and save the displayed figure(s) at the temperature(s) you specified.');\n    disp(part2);\nend\n%Write a CSV file of all CTE data\nif Want_A_Printout==1\n    [EVang1,EVang2,EVang3]=EVAngles(V,D,ConMat,Temps_to_be_Analyzed,[aplaneorient;bplaneorient;cplaneorient],lsfits,HKL1);\n    fidpath=strcat(outputsavelocation,Printout_Filename,'.csv');\n    fid2=fopen(fidpath,'wt');\n    fprintf(fid2,'Temp,CTE(11),CTE(12),CTE(13),CTE(21),CTE(22),CTE(23),CTE(31),CTE(32),CTE(33),Eig1,Eig2,Eig3,Beta-V,Alpha-V,Ev1(1),Ev1(2),Ev1(3),Ev2(1),Ev2(2),Ev2(3),Ev3(1),Ev3(2),Ev3(3),Eig1Angle,Eig2Angle,Eig3Angle\\n');\n    for n=1:NumCalcs\n        fprintf(fid2,'%4.4f,',Temps_to_be_Analyzed(n));\n        for nn=1:3\n            for nnn=1:3\n                fprintf(fid2,'%d,',Tensor(nn,nnn,n));\n            end\n            if(nn==3)\n                BetaV=D(1,n)+D(2,n)+D(3,n);\n                AlphaV=BetaV/3;\n                fprintf(fid2,'%d,',D(1,n),D(2,n),D(3,n),BetaV,AlphaV,V(1,1,n),V(2,1,n),V(3,1,n),V(1,2,n),V(2,2,n),V(3,2,n),V(1,3,n),V(2,3,n),V(3,3,n),EVang1(n),EVang2(n),EVang3(n));\n                fprintf(fid2,'\\n');\n            end\n        end\n    end\n    %If a figure is being plotted in this run, add those data to the file.\n    if Want_Figures==1\n        fprintf(fid2,'\\nData for Figures\\n');\n        for figctr=1:NumFigs;\n            fprintf(fid2,'%4.4f,',Figure_Temps(figctr));\n            for nn=1:3\n                for nnn=1:3\n                    fprintf(fid2,'%d,',TensorFigs(nn,nnn,figctr));\n                end\n                if(nn==3)\n                    BetaVfig=DFig(1,figctr)+DFig(2,figctr)+DFig(3,figctr);\n                    AlphaVfig=BetaVfig/3;\n      \t\t            fprintf(fid2,'%d,',DFig(1,figctr),DFig(2,figctr),DFig(3,figctr),BetaVfig,AlphaVfig,VFig(1,1,figctr),VFig(2,1,figctr),VFig(3,1,figctr),VFig(1,2,figctr),VFig(2,2,figctr),VFig(3,2,figctr),VFig(1,3,figctr),VFig(2,3,figctr),VFig(3,3,figctr));\n                    fprintf(fid2,'\\n');\n                end\n            end\n        end\n    end\n    fclose(fid2);\n    part3=sprintf('Data File created as %s',fidpath);\n    disp(part3);\nend\nif Want_2D_Figures==1\n    twodvals=EllipseWrap(Tensor,ConMat,Temps_to_be_Analyzed,aorient,borient,corient,lsfits,Xscreensize,Yscreensize,HKL2);\n    part4=sprintf('2D Cross-Section Figures Plotted.');\n    disp(part4);\n    if Output_2D_Figure_Data==1\n        WriteTwoDCSV(twodvals,Temps_to_be_Analyzed,strcat(outputsavelocation,Output_2D_Filename));\n        part4a=sprintf('2D X & Y Values Output to %s.csv',strcat(outputsavelocation,Output_2D_Filename));\n        disp(part4a);\n    end\nend\nif Want_Eig_Plot==1\n    PlotEigenvalues(Tensor,Temps_to_be_Analyzed,Xscreensize,Yscreensize);\n    part5=sprintf('Eigenvalue Figure Plotted.  Please save it.');\n    disp(part5);\nend\nif Want_HKLorUVW_Expansion_Plot==1\n%need to resolve <1 HKL/UVW issues\n    if HKL2==1\n        inhkl='uvw';\n        inhkl2=' uvw';\n        INHKL='UVW';\n    else\n        inhkl='hkl';\n        inhkl2=' hkl';\n        INHKL='HKL';\n    end\n    t1=aorient;\n    string1=num2str(t1);\n    t2=borient;\n    string2=num2str(t2);\n    t3=corient;\n    string3=num2str(t3);\n    point='p';\n    if mod(abs(t1),1)<1 && mod(abs(t1),1)>0\n        stuff1=t1;\n        if abs(stuff1)<1\n            stuff1=0;\n        end\n        string1=sprintf('%1.0f%s%2.0f',stuff1,point,mod(abs(t1),1)*100);\n    end\n    if mod(abs(t2),1)<1 && mod(abs(t2),1)>0\n        stuff2=t2;\n        if abs(stuff2)<1\n            stuff2=0;\n        end\n        string2=sprintf('%1.0f%s%2.0f',stuff2,point,mod(abs(t2),1)*100);\n    end\n    if mod(abs(t3),1)<1 && mod(abs(t3),1)>0\n        stuff3=t3;\n        if abs(stuff3)<1\n            stuff3=0;\n        end\n        string3=sprintf('%1.0f%s%2.0f',stuff3,point,mod(abs(t3),1)*100);\n    end\n    HKLorUVW=[aorient;borient;corient];\n    HKLvals=HKLExpansion(ConMat,Tensor,HKLorUVW,Temps_to_be_Analyzed,Xscreensize,Yscreensize,lsfits,HKL2);\n    part6=sprintf(strcat(INHKL,' Expansion Figure Plotted.  Please Save it.'));\n    disp(part6);\n    if Save_HKL_Expansion_Printout==1\n    fid3=fopen(strcat(outputsavelocation,HKL_Filename_Prefix,'-',inhkl,'_',string1,'_',string2,'_',string3,'_Expansion.csv'),'wt');\n    fprintf(fid3,strcat('Thermal Expansion along: ',inhkl2,'=[',num2str(HKLorUVW(1)),';',num2str(HKLorUVW(2)),';',num2str(HKLorUVW(3)),'] direction.\\n'));\n    fprintf(fid3,strcat('T(',char(176),'C),alpha_hkl\\n'));\n    for counter=1:length(HKLvals)\n        fprintf(fid3,'%4.4f,',Temps_to_be_Analyzed(counter));\n        fprintf(fid3,'%d\\n',HKLvals(counter));\n    end\n    fclose(fid3);\n    part7=sprintf(strcat(INHKL,' Expansion printout written as:'));\n\n    fpathhkl=strcat(outputsavelocation,HKL_Filename_Prefix,'-',inhkl,'_',string1,'_',string2,'_',string3,'_Expansion.csv');\n    disp(part7);\n    disp(fpathhkl);\n    end\nend\npart8=sprintf('Thanks for using CTERun!');\ndisp(part8);\nDone=0;"("Input_File_Directory_Location"=w216, "Want_A_Movie"=w215, "Want_Figures"=w214, "Want_A_Printout"=w211, "Want_Eig_Plot"=w213, "Want_2D_Figures"=w212, "Movie_File_Name"="Movie File Name", "Printout_Filename"="CSV File Name", "Figure_Temps"="Figure Temperature (C)", "aorient"=w199, "borient"=w198, "corient"=w197, "aplaneorient"=w196, "bplaneorient"=w195, "cplaneorient"=w194, "Xscreensize"=w193, "Yscreensize"=w192, "HKL1"=w203, "HKL2"=w202, "Want_HKLorUVW_Expansion_Plot"=w200, "fps"="Movie FPS", "Output_2D_Figure_Data"=w190, "Output_2D_Filename"="2D Figure CSV File Name", "Save_HKL_Expansion_Printout"=w187, "HKL_Filename_Prefix"="hkl (or uvw) Expansion CSV Filename") -> ("Done"=w205:dbl)  [unwired: 1 in, 1 out]
        n145 = Not Equal To 0?(x=w205) -> (x != 0?=w204:bool)
        n146 = local write "BUSY"(w204) -> ()
        "BUSY" <- w206
      }
    }
  }
